vi "PC_Pub_imgFile retrieveImg.vi"(8 "error in (no error)":errorcluster, 11 "imgFile in":refnum<class "PC_Pub_imgFile.lvclass">) -> (0 "error out":errorcluster, 3 "imgFile out":refnum<class "PC_Pub_imgFile.lvclass">)   [LabVIEW 2018, in "PC_Pub_imgFile.lvclass"]
uses:
  PC_Pub_imgFile.lvclass
  PC_Pub_imgFile.lvclass/PC_Pub_imgFile.ctl
  <vilib>/nisyscfg/nisyscfg.lvlib
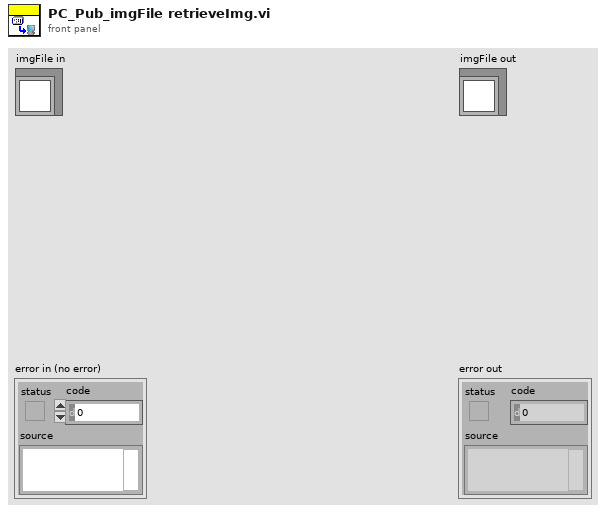
[diagram p1: front panel]
types:
  T1 = typedef "nisyscfg.lvlib/Software 1.2.ctl" = cluster{"title":string, "description":string, "ID":string, "version":string, "component type":T2}
  T2 = typedef "nisyscfg.lvlib/Component Type.ctl" = u32
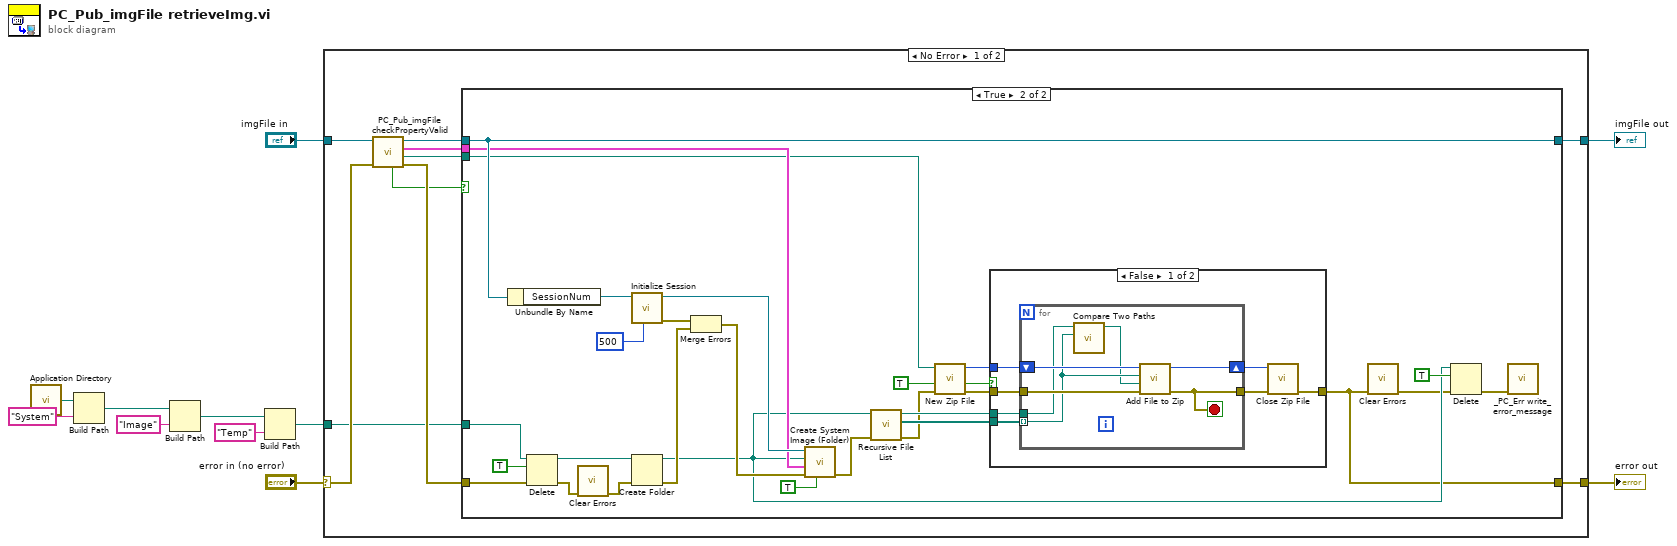
[diagram p0: block diagram]
diagram:
  n1 = call <vilib>:"Application Directory.vi"() -> ("Application Directory"=w6:path)
  n2 = Build Path(base path=w6, name or relative path="System") -> (appended path=w5:path)
  n3 = Build Path(base path=w5, name or relative path="Image") -> (appended path=w7:path)
  n4 = Build Path(base path=w7, name or relative path="Temp") -> (appended path=w1:path)
  n5 = case shown="No Error" "error in (no error)" {
    selector: "error in (no error)" -> [w18 w69]
    tunnel: [w21 w69] -> w11
    tunnel: [w16 w68] -> w9
    tunnel: "imgFile in" -> [w20 w68]
    tunnel: w1 -> [w12 _]
    frame No Error {
      n6 = call "PC_Pub_imgFile checkPropertyValid.vi"("error in (no error)"=w18, "imgFile in"=w20) -> ("error out"=w17:errorcluster, "appended path"=w13:path, "Image Metadata in"=w14:T1, "imgFile out"=w19:refnum<class "PC_Pub_imgFile.lvclass">, "valid"=w15:bool)  [unwired: 5 in]
      n7 = case shown="True" w15 {
        tunnel: [w23 w26] -> w21
        tunnel: w19 -> [w22 w33]
        tunnel: w17 -> [w23 w34]
        tunnel: [w22 w33] -> w16
        tunnel: w14 -> [_ w32]
        tunnel: w13 -> [_ w31]
        tunnel: w12 -> [_ w28]
        frame False {
        }
        frame True {
          n8 = Unbundle By Name(w33) -> ("SessionNum"=w48:refnum<k21>)
          n9 = Delete(path (use dialog)=w28, entire hierarchy (F)=TRUE, error in=w34) -> (deleted path=w51:path, error out=w50:errorcluster)  [unwired: 2 in, 1 out]
          n10 = call <vilib>:"Clear Errors.vi"("error in (no error)"=w50) -> ("error out"=w49:errorcluster)  [unwired: 5 in, 1 out]
          n11 = call <vilib>:"Initialize Session.vi"("Connect Timeout (4000 ms)"=u32 500, "Target (localhost)"=w48) -> ("error out"=w45:errorcluster, "Session out"=w47:refnum<k21>)  [unwired: 8 in]
          n12 = Create Folder(path (use dialog)=w51, error in=w49) -> (created path=w30:path, error out=w44:errorcluster)  [unwired: 1 in, 1 out]
          n13 = Merge Errors(w45, w44) -> (w43:errorcluster)
          n14 = call <vilib>:"Create System Image (Folder).vi"("Overwrite (F)"=TRUE, "error in (no error)"=w43, "Image Metadata in"=w32, "Destination Folder"=w30, "Session in"=w47) -> ("error out"=w36:errorcluster)  [unwired: 4 in, 2 out]
          n15 = call <vilib>:"Recursive File List.vi"("error in (no error)"=w36, "Folder Path"=w30) -> ("error out"=w35:errorcluster, "All Files in Dir"=w42:path[], "dup Folder Path"=w41:path)  [unwired: 1 in, 6 out]
          n16 = call <vilib>:"New Zip File.vi"("error in (no error)"=w35, "confirm overwrite? (F)"=TRUE, "target"=w31) -> ("error out"=w40:errorcluster, "cancelled"=w25:bool, "zip file out"=w39:i64)  [unwired: 2 out]
          n17 = case shown="False" w25 {
            tunnel: w42 -> [w59 _]
            tunnel: w41 -> [w58 _]
            tunnel: w40 -> [w55 w67]
            tunnel: w39 -> [w54 _]
            tunnel: [w53 w67] -> w26
            frame False {
              n18 = for {
                shift-right: [w65] -> w56
                shift-left: w54 -> [w66]
                tunnel: w55 -> [w64]
                tunnel: [w63] -> w57
                tunnel: w58 -> [w62]
                tunnel: w59 -> [w61] mode=indexing
                stop <- w63 stop-if-true
                n19 = call <vilib>:"Compare Two Paths.vi"("Path 2"=w61, "Path 1"=w62) -> ("Relative Path from 1 to 2"=w60:path)  [unwired: 1 in, 8 out]
                n20 = call <vilib>:"Add File to Zip.vi"("error in (no error)"=w64, "destination path in zip"=w60, "source file path"=w61, "zip file in"=w66) -> ("error out"=w63:errorcluster, "zip file out"=w65:i64)  [unwired: 6 out]
              }
              n21 = call <vilib>:"Close Zip File.vi"("error in (no error)"=w57, "zip file in"=w56) -> ("error out"=w53:errorcluster)  [unwired: 1 in, 4 out]
            }
            frame True {
            }
          }
          n22 = call <vilib>:"Clear Errors.vi"("error in (no error)"=w26) -> ("error out"=w29:errorcluster)  [unwired: 5 in, 1 out]
          n23 = Delete(path (use dialog)=w30, entire hierarchy (F)=TRUE, error in=w29) -> (error out=w27:errorcluster)  [unwired: 2 in, 2 out]
          n24 = call "_PC_Err write_error_message.vi"("error in"=w27) -> ()  [unwired: 10 in, 1 out]
        }
      }
    }
    frame Error {
    }
  }
  "error out" <- w11
  "imgFile out" <- w9
